vi "Bug man temp globals.vi"() -> ()   [LabVIEW 2019]
doc: "Thise are the global variables for the bug experiment.\n\nThe \"exec\" cluster is under executive control, all other variables are under control of the DAQ state machine.\n\nPaul K Dxion\nP3600\nCSUSB Physics"
uses:
  typedefs/temp cont cluster.ctl
  typedefs/temp exec cluster.ctl
  typedefs/temp mode enum.ctl
  typedefs/temp indicator.ctl
  typedefs/temp cont utility.ctl
panel:
  in  "T cont":T1={"exec"={"T mode"=enum."Listening to exec", "log"=FALSE, "thermistor"=enum."solo"}, "T status"={"Temp"=0.0}, "utility"={"meas index"=0, "wait (ms)"=300, "therm volt"=0.0, "t T hist"=[]}} {"utility"."therm volt" format="%_6g"; "T status"."Temp" format="%_6g"}
  # "exec, wait, and T params are under exec control"
  # "T status and the voltages are under DAQ state machine control"
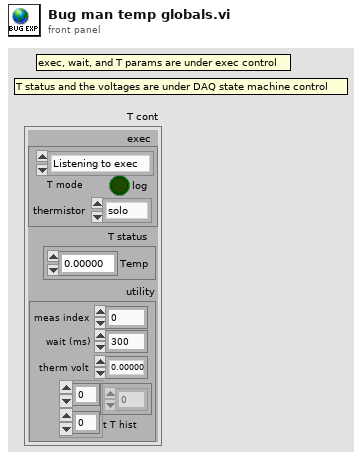
[diagram p1: front panel]
types:
  T1 = typedef "temp cont cluster.ctl" = cluster{"exec":T2, "T status":T4, "utility":T5}
  T2 = typedef "temp exec cluster.ctl" = cluster{"T mode":T3, "log":bool, "thermistor":enum16{"solo", "bug"}}
  T3 = typedef "temp mode enum.ctl" = enum16{"Setting up", "Listening to exec", "Exit"}
  T4 = typedef "temp indicator.ctl" = cluster{"Temp":dbl}
  T5 = typedef "temp cont utility.ctl" = cluster{"meas index":i32, "wait (ms)":i32, "therm volt":dbl, "t T hist":dbl[][]}
diagram:
